vi "Set Overload Protection Timeout.vi"(8 "error in (no error)":errorcluster, 10 "Timeout Value (1.0 s)":dbl=1.0 format="%.4f", 11 "VISA resource name":refnum<visa-resource-name>) -> (0 "error out":errorcluster, 3 "VISA resource name out":refnum<visa-resource-name>)   [LabVIEW 2011, in "Fluke 5XXX Series Multicalibrators.lvlib"]
doc: "This VI sets the OPERATE time limit for the OVERLD mode signal. The Calibrator automatically returns to STANDBY if the UUT protection trips within this interval or at the end of this interval if the protection has not tripped.\n\nNote:\n\nThis VI is available only for instrument models 5500A and 5520A with oscilloscope option SC600 (SC1100)."
uses:
  Fluke 5XXX Series Multicalibrators.lvlib
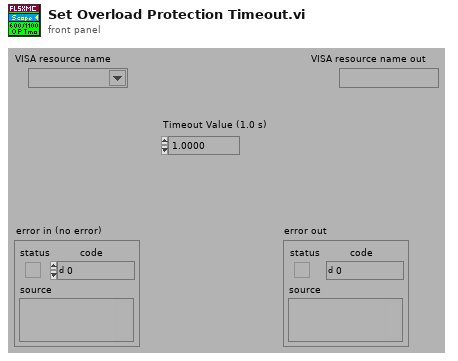
[diagram p1: front panel]
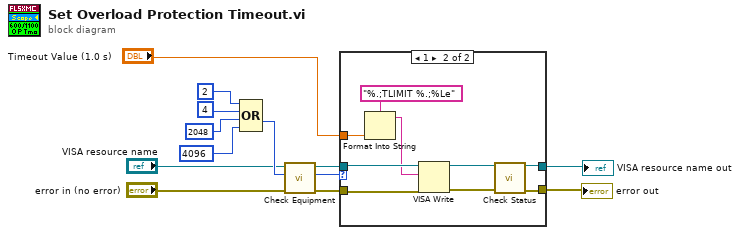
[diagram p0: block diagram]
diagram:
  n1 = Compound Arithmetic op=OR(2 ("Numeric"), 4 ("Numeric"), 2048 ("Numeric"), 4096 ("Numeric")) -> (w7:i32)
  n2 = call "Check Equipment.vi"("error in (no error)"="error in (no error)", "Bit Mask"=w7, "VISA resource name"="VISA resource name") -> ("error out"=w10:errorcluster, "Present?"=w9:u32, "VISA resource name out"=w8:refnum<visa-resource-name>)  [unwired: 6 in]
  n3 = case shown="1" w9 {
    tunnel: [w14 w22] -> w2
    tunnel: w10 -> [w15 w24]
    tunnel: w8 -> [w14 w18]
    tunnel: [w15 w23] -> w3
    tunnel: "Timeout Value (1.0 s)" -> [_ w16]
    frame 0, Default {
    }
    frame 1 {
      n4 = Format Into String(format string="%.;TLIMIT %.;%Le", w16) -> (resulting string=w17:string)  [unwired: 2 in, 1 out]
      n5 = VISA Write(VISA resource name=w18, write buffer=w17, error in (no error)=w24) -> (VISA resource name out=w20:refnum<visa-resource-name>, error out=w21:errorcluster)  [unwired: 1 out]
      n6 = call "Check Status.vi"("VISA resource name"=w20, "error in (no error)"=w21) -> ("VISA resource name out"=w22:refnum<visa-resource-name>, "error out"=w23:errorcluster)  [unwired: 12 in]
    }
  }
  "VISA resource name out" <- w2
  "error out" <- w3
